vi "Read All Instruments.vi"(1 "Instrument Array In":T1[](array[typedef]) {"Private"."Offset" format="%^_3e"; "Private"."Scale Factors" format="%^_3e"}) -> (2 "Data Array":dbl[](array[numeric]) format="%_6e", 3 "Instrument Array Out":T1[](array[typedef]) {"Private"."Offset" format="%^_3e"; "Private"."Scale Factors" format="%^_3e"}, 4 "Time (mS)":dbl[](array[numeric]), 5 "Instrument Stop":bool[](array[boolean]))   [LabVIEW 2025]
doc: "Author: Scott Hannahs <sth@magnet.fsu.edu>\n\nThis software is licensed for use under the “MIT License\"\nCopyright (c) 2025 Scott Hannahs, sth@sth@magnet.sthnet.net\n\nPermission is hereby granted, free of charge, to any person obtaining a copy of this software and associated documentation files (the \"Software\"), to deal in the Software without restriction, including without limitation the rights to use, copy, modify, merge, publish, distribute, sublicense, and/or sell copies of the Software, and to permit persons to whom the Software is furnished to do so, subject to the following conditions: The above copyright notice and this permission notice shall be included in all copies or substantial portions of the Software.\n\nTHE SOFTWARE IS PROVIDED \"AS IS\", WITHOUT WARRANTY OF ANY KIND, EXPRESS OR IMPLIED, INCLUDING BUT NOT LIMITED TO THE WARRANTIES OF MERCHANTABILITY, FITNESS FOR A PARTICULAR PURPOSE AND NONINFRINGEMENT. IN NO EVENT SHALL THE AUTHORS OR COPYRIGHT HOLDERS BE LIABLE FOR ANY CLAIM, DAMAGES OR OTHER LIABILITY, WHETHER IN AN ACTION OF CONTRACT, TORT OR OTHERWISE, ARISING FROM, OUT OF OR IN CONNECTION WITH THE SOFTWARE OR THE USE OR OTHER DEALINGS IN THE SOFTWARE."
uses:
  Sub Controls/Instrument Properties.ctl
  Sub Controls/Public.ctl
  Sub Controls/Private.ctl
  Sub Controls/Instrument Ref.ctl
  Sub Controls/SystemCheckBox-resize.ctl
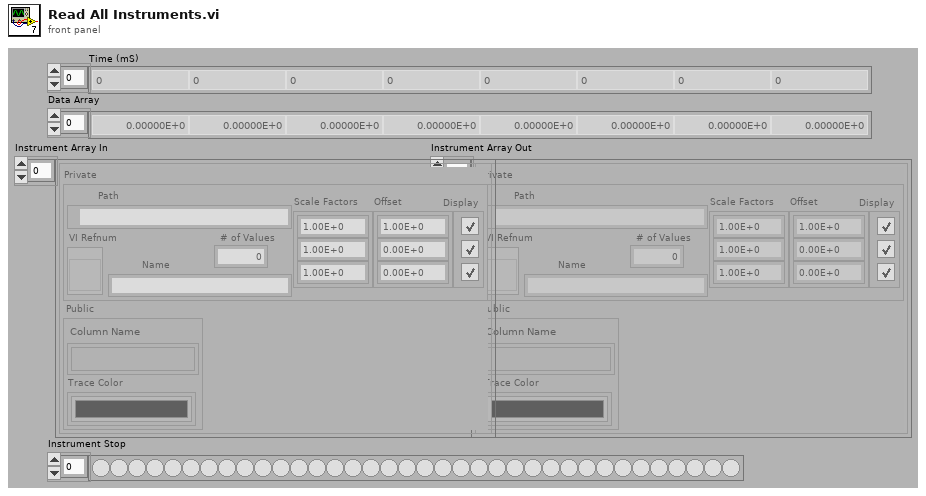
[diagram p1: front panel]
types:
  T1 = typedef "Instrument Properties.ctl" = cluster{"Public":T2, "Private":T3}
  T2 = typedef "Public.ctl" = cluster{"Column Name":string[], "Trace Color":u32[]}
  T3 = typedef "Private.ctl" = cluster{"Path":path, "VI Refnum":T4, "Name":string, "# of Values":i32, "Scale Factors":dbl[], "Display":T5[], "Offset":dbl[]}
  T4 = typedef "Instrument Ref.ctl" = refnum<vi>
  T5 = typedef "SystemCheckBox-resize.ctl" = bool
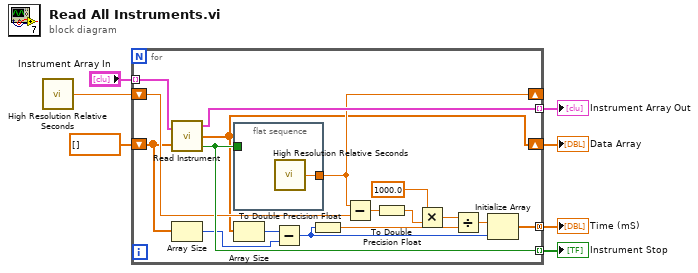
[diagram p0: block diagram]
diagram:
  n1 = call <vilib>:"High Resolution Relative Seconds.vi"() -> ("relative seconds"=w2:dbl)
  n2 = for {
    tunnel: "Instrument Array In" -> [w24] mode=indexing
    tunnel: [w23] -> w6 mode=indexing
    shift-right: [w17] -> w3
    shift-left: dbl[] [] ("Array 2") -> [w12]
    tunnel: [w22] -> w7 mode=indexing
    tunnel: [w19] -> w1 mode=concatenating
    shift-right: [w20] -> _
    shift-left: w2 -> [w21]
    n3 = call "Read Instrument.vi"("Instrument Prop In"=w24, "Array In"=w12) -> ("Instrument Prop Out"=w23:T1, "Array Out"=w17:dbl[], "Stop"=w22:bool)
    n4 = Array Size(array=w12) -> (size(s)=w10:i32)
    n5 = flat-sequence {
      tunnel: w22 -> [_]
      tunnel: [w25] -> w20
      frame #0 {
        n6 = call <vilib>:"High Resolution Relative Seconds.vi"() -> ("relative seconds"=w25:dbl)
      }
    }
    n7 = Array Size(array=w17) -> (size(s)=w15:i32)
    n8 = Subtract(x=w15, y=w10) -> (x-y=w11:i32)
    n9 = To Double Precision Float(number=w11) -> (double precision float=w13:dbl)
    n10 = Subtract(x=w20, y=w21) -> (x-y=w18:dbl)
    n11 = To Double Precision Float(number=w18) -> (double precision float=w14:dbl)
    n12 = Multiply(x=1000.0, y=w14) -> (x*y=w9:dbl)
    n13 = Divide(x=w9, y=w13) -> (x/y=w16:dbl)
    n14 = Initialize Array(w16, w11) -> (w19:dbl[])
  }
  "Data Array" <- w3
  "Instrument Stop" <- w7
  "Instrument Array Out" <- w6
  "Time (mS)" <- w1
